vi "ALU.vi"(0 "zx":bool, 1 "x":bool[](array[boolean])=[FALSE, FALSE, FALSE, FALSE, FALSE, FALSE, FALSE, FALSE, FALSE, FALSE, FALSE, FALSE, FALSE, FALSE, FALSE, FALSE], 4 "y":bool[](array[boolean])=[FALSE, FALSE, FALSE, FALSE, FALSE, FALSE, FALSE, FALSE, FALSE, FALSE, FALSE, FALSE, FALSE, FALSE, FALSE, FALSE], 6 "nx":bool, 8 "zy":bool, 10 "ny":bool, 12 "f":bool, 14 "no":bool) -> (9 "zr":bool, 11 "ng":bool, 17 "out":bool[](array[boolean]))   [LabVIEW 2014]
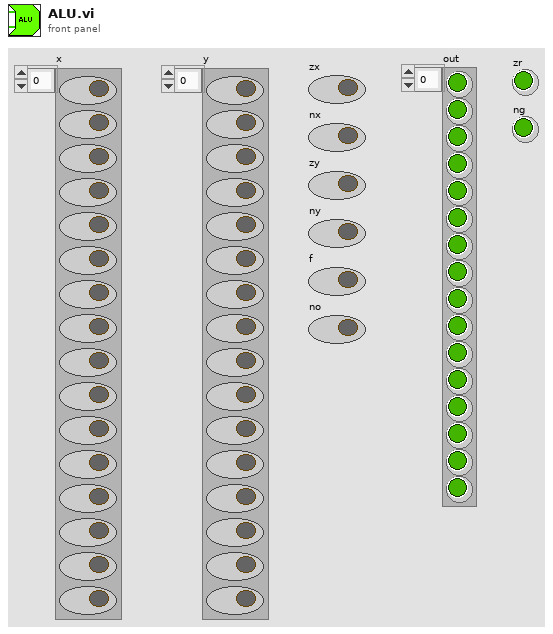
[diagram p1: front panel]
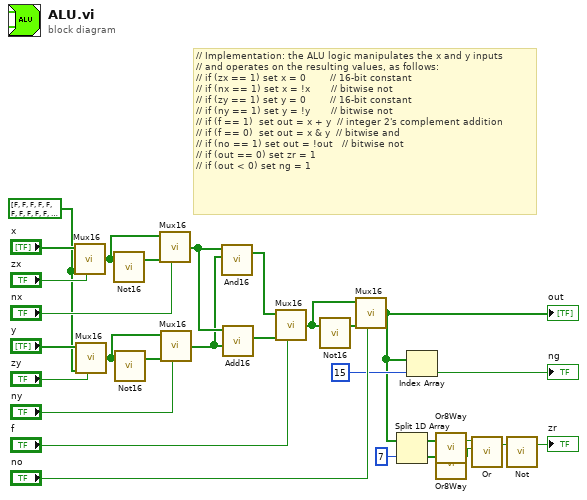
[diagram p0: block diagram]
diagram:
  w19 = bool[] [FALSE, FALSE, FALSE, FALSE, FALSE, FALSE, FALSE, FALSE, FALSE, FALSE, FALSE, FALSE, FALSE, FALSE, FALSE, FALSE]
  # "// Implementation: the ALU logic manipulates the x and y inputs\n// and operates on the resulting values, as follows:\n// if (zx == 1) set x = 0        // 16-bit constant\n// if (nx == 1) set x = !x       // bitwise not\n// if (zy == 1) set y = 0        // 16-bit constant\n// if (ny == 1) set y = !y       // bitwise not\n// if (f == 1)  set out = x + y  // integer 2's complement addition\n// if (f == 0)  set out = x & y  // bitwise and\n// if (no == 1) set out = !out   // bitwise not\n// if (out == 0) set zr = 1\n// if (out < 0) set ng = 1"
  n1 = call "Mux16.vi"("a"="x", "sel"="zx", "b"=w19) -> ("out"=w26:bool[])  [unwired: 5 in]
  n2 = call "Mux16.vi"("a"="y", "sel"="zy", "b"=w19) -> ("out"=w24:bool[])  [unwired: 5 in]
  n3 = call "Not16.vi"("in"=w26) -> ("out"=w27:bool[])  [unwired: 2 in]
  n4 = call "Not16.vi"("in"=w24) -> ("out"=w23:bool[])  [unwired: 2 in]
  n5 = call "Mux16.vi"("a"=w26, "sel"="nx", "b"=w27) -> ("out"=w18:bool[])  [unwired: 5 in]
  n6 = call "Mux16.vi"("a"=w24, "sel"="ny", "b"=w23) -> ("out"=w17:bool[])  [unwired: 5 in]
  n7 = call "And16.vi"("b"=w17, "a"=w18) -> ("out"=w15:bool[])  [unwired: 3 in]
  n8 = call "Add16.vi"("b"=w17, "a"=w18) -> ("out"=w14:bool[])  [unwired: 6 in]
  n9 = call "Mux16.vi"("a"=w15, "sel"="f", "b"=w14) -> ("out"=w12:bool[])  [unwired: 5 in]
  n10 = call "Not16.vi"("in"=w12) -> ("out"=w13:bool[])  [unwired: 2 in]
  n11 = call "Mux16.vi"("a"=w12, "sel"="no", "b"=w13) -> ("out"=w8:bool[])  [unwired: 5 in]
  "out" <- w8
  n12 = Split 1D Array(array=w8, index=7) -> (first subarray=w7:bool[], second subarray=w6:bool[])
  n13 = Index Array(array=w8, index=15) -> (element=→"ng":bool)
  n14 = call "Or8Way.vi"("in"=w7) -> ("out"=w5:bool)  [unwired: 2 in]
  n15 = call "Or8Way.vi"("in"=w6) -> ("out"=w4:bool)  [unwired: 2 in]
  n16 = call "Or.vi"("b"=w4, "a"=w5) -> ("out"=w3:bool)  [unwired: 3 in]
  n17 = call "Not.vi"("in"=w3) -> ("out"=→"zr":bool)  [unwired: 2 in]
